vi "Destroy.vi"(0 "reference in":refnum<class "DAQ_Base.lvclass">, 5 "error in (no error)":errorcluster) -> (14 "reference out":refnum<class "DAQ_Base.lvclass">, 19 "error out":errorcluster)   [LabVIEW 2020, in "DAQ.lvlib" / "DAQ_Base.lvclass"]
uses:
  DAQ_Base.lvclass
  <vilib>/addons/_AddQ/G#Object/G#Object.lvclass
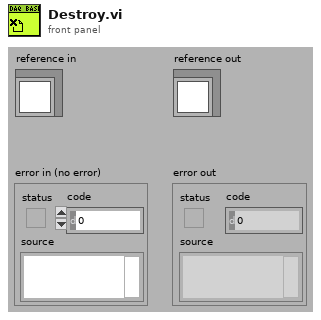
[diagram p1: front panel]
types:
  T1 = typedef "DAQ.lvlib/DAQ_Base.lvclass/ObjectAttributes.ctl" = cluster{"MyAttribute":dbl, "RootPath":path, "DAQSettings":T2, "DaqCollector":cluster{"CollectDataQueue":refnum<queue>, "ArryDataCollectorChannel":T8[], "RealTimeValues":dbl[]}, "CollectorChannelEnable":bool[]}
  T2 = typedef "DAQ.lvlib/DAQ_Base.lvclass/DAQSettings.ctl" = cluster{"SampleSettings":T3, "AI_ChannelSettings":T4, "AO_ChannelSettings":T6, "Cnt_ChannelSettings":T7}
  T3 = typedef "DAQ.lvlib/DAQ_Base.lvclass/SampleSettings.ctl" = cluster{"samples per channel":i32, "SampleRate":dbl, "TansMaxLength":dbl, "ReadTimeOut":dbl, "时钟源":tag}
  T4 = typedef "DAQ.lvlib/DAQ_Base.lvclass/AI_ChannelSettings.ctl" = cluster{"AI_SettingsArry":cluster{"DeviceName":tag, "physical channels":tag, "AssignName":string, "输入信号类型":T5, "Max_value":dbl, "Min_value":dbl, "单位":i32, "shunt resistor location":i32, "external shunt resistor value":dbl, "标定系数":cluster{"Scale":dbl, "Offset":dbl}}[]}
  T5 = typedef "AI信号类型.ctl" = i32
  T6 = typedef "DAQ.lvlib/DAQ_Base.lvclass/AO_ChannelSettings.ctl" = cluster{"布尔":bool}
  T7 = typedef "DAQ.lvlib/DAQ_Base.lvclass/Cnt_ChannelSettings.ctl" = cluster{"Cnt_ChannelSettings":cluster{"类型":enum16{"Linear", "Rotate"}, "CounterNbr":tag, "AssignName":string, "单位":u16, "decoding type":u16, "PPR_DistancePerPulse":dbl, "Initial Position ":dbl, "z index enable":bool, "z index phase":i32, "source":tag}[]}
  T8 = typedef "DAQ.lvlib/DAQ_Base.lvclass/DataCollector.ctl" = cluster{"DataCollectArry":dbl[][], "Update":bool}
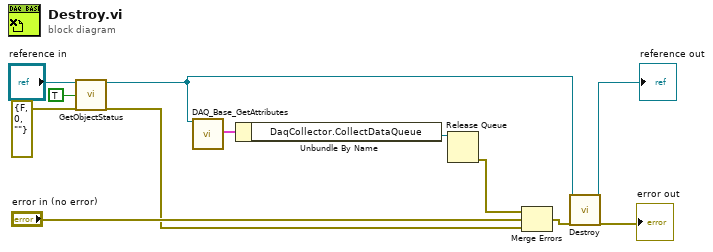
[diagram p0: block diagram]
diagram:
  n1 = call-dynamic "GetObjectStatus.vi"("reference in"="reference in", "simple info (F)"=TRUE ("simple info"), "error in (no error)"=errorcluster {"status"=FALSE, "code"=0, "source"=""}) -> ("reference out"=w4:refnum<class "DAQ_Base.lvclass">, "error out"=w5:errorcluster)  [unwired: 5 in, 10 out]
  n2 = call "DAQ_Base_GetAttributes.vi"("reference in"=w4) -> ("attributes"=w3:T1)  [unwired: 15 in, 3 out]
  n3 = Unbundle By Name(w3) -> ("DaqCollector.CollectDataQueue"=w2:refnum<queue>)
  n4 = Release Queue(queue=w2) -> (error out=w1:errorcluster)  [unwired: 2 in, 2 out]
  n5 = Merge Errors(w1, "error in (no error)", w5) -> (w11:errorcluster)
  n6 = call-parent "Destroy.vi"("reference in"=w4, "error in (no error)"=w11) -> ("reference out"=→"reference out":refnum<class "DAQ_Base.lvclass">, "error out"=→"error out":errorcluster)  [unwired: 16 in]
